vi "STM Comm Lookup Table_Initialize.vi"(8 "error in (no error)":errorcluster) -> (0 "error out":errorcluster {"code" min=0 max=0}, 3 "vi reference":T1)   [LabVIEW 2015, in "Control Addon Engine.lvlib" / "STM.lvlib"]
uses:
  STM.lvlib
  STM Comm Lookup Table_Ref.ctl
  <userlib>/STM/Connection Manager/TCP/stm_TCPConnectionMethod.ctl
  STM TCP Connection Manager.vi
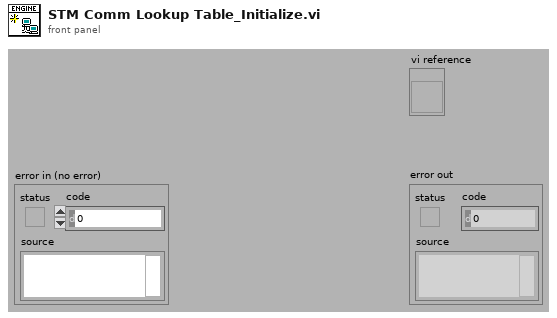
[diagram p1: front panel]
types:
  T1 = typedef "Control Addon Engine.lvlib/STM.lvlib/STM Comm Lookup Table_Ref.ctl" = refnum<vi>
  T2 = typedef "stm_TCPConnectionMethod.ctl" = enum16{"Initialize", "Add Connection", "Set Properties", "Get Connection(s)", "Remove Connection", "Remove All Connections", "Get Connection Count"}
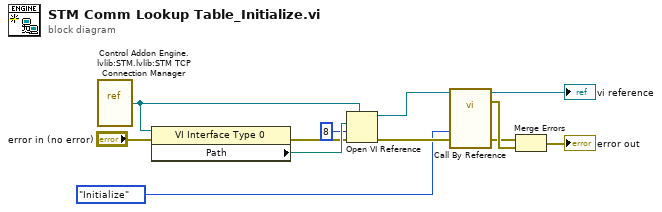
[diagram p0: block diagram]
diagram:
  n1 = vi-ref "Control Addon Engine.lvlib:STM.lvlib:STM TCP Connection Manager.vi"() -> (w2:refnum<vi>)
  n2 = property class="VI Interface Type 0"(reference=w2, error in="error in (no error)") -> (error out=w10:errorcluster, "Path"=w12:path)  [unwired: 1 out]
  n3 = Open VI Reference(type specifier VI Refnum (for type only)=w2, vi path=w12, options=8, error in (no error)=w10) -> (vi reference=w9:refnum<vi>, error out=w5:errorcluster)  [unwired: 2 in]
  n4 = call-by-ref "?"(reference=w9, "error in (no error)"=w5, "Method"=stm_TCPConnectionMethod."Initialize") -> (reference out=→"vi reference":refnum<vi>, error out=w8:errorcluster, 0:"error out"=w4:errorcluster)  [unwired: 5 in, 5 out]
  n5 = Merge Errors(w4, w8) -> (→"error out":errorcluster)
